vi "Add To DAQmx Task.vi"(6 "Ignore Cal? (F)":bool, 7 "Resistance in":refnum<class "Resistance.lvclass">, 8 "error in (no error)":errorcluster, 9 "Scale Name":string, 10 "Chassis Name":string, 11 "task in":refnum<k21>) -> (0 "error out":errorcluster, 2 "Phys Chan Added":string, 3 "task out":refnum<k21>)   [LabVIEW 2018, in "Measurement Channels.lvlib" / "Resistance.lvclass"]
uses:
  Resistance.lvclass
  C:/Users/Jeff Tipps/Documents/DAQMan/source/Classes/Measurements/Class Channel/Channel.lvclass
  Resistance.lvclass/Resistance.ctl
  Class Channel/Read ChanName.vi
  Class Channel/Read Alias.vi
  Class Channel/Read Scale.vi
  Class Channel/Read Offset.vi
  Class Channel/Read Unit_EU.vi
  <vilib>/DAQmx/create/scale.llb/DAQmx Create Scale (Linear).vi
  <vilib>/DAQmx/create/channels.llb/DAQmx Create Channel (AI-Resistance).vi
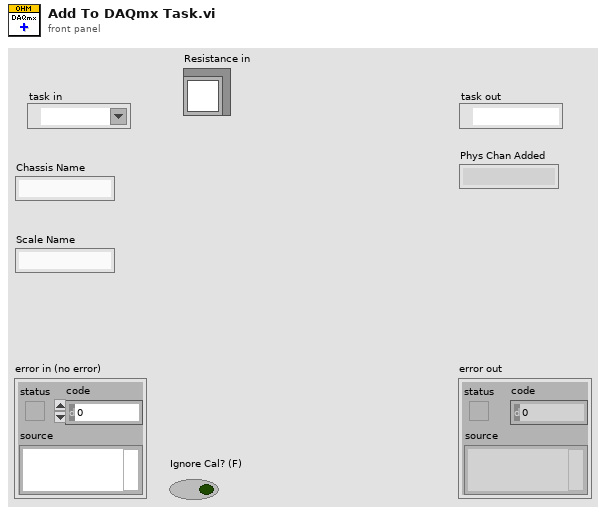
[diagram p1: front panel]
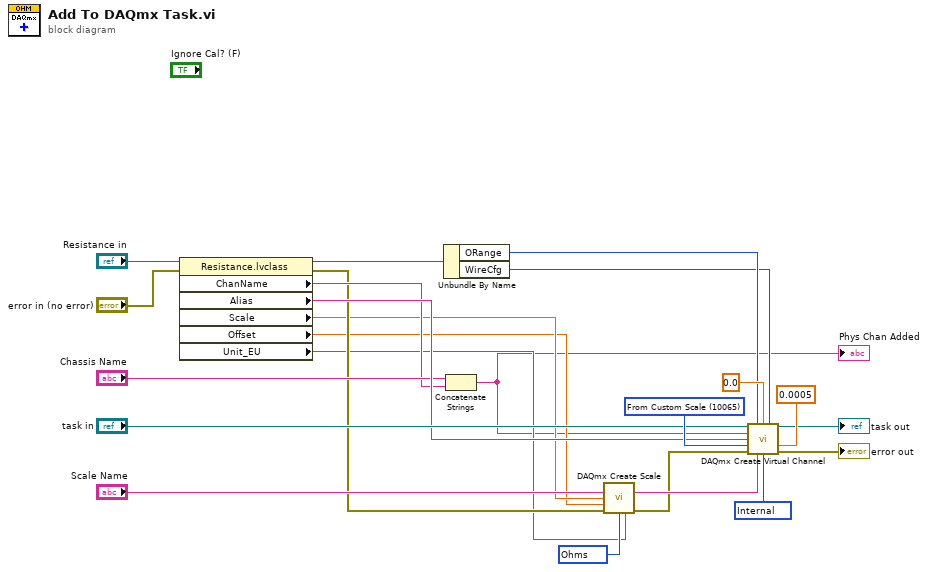
[diagram p0: block diagram]
diagram:
  w22 = 10384 items=["Volts"=10348, "Amps"=10342, "Deg F"=10144, "Deg C"=10143, "Deg R"=10145, "Kelvins"=10325, "Strain"=10299, "Ohms"=10384, "Hz"=10373, "Seconds"=10364, "Meters"=10219, "Inches"=10379, "Degrees"=10146, "Radians"=10273, "Ticks"=10304, "g"=10186, "m/s^2"=12470, "m/s"=15959, "in/s"=15960, "Pascals"=10081, "Newtons"=15875, "Pounds"=15876, "kgf"=15877, "psi"=15879, "bar"=15880, "Nm"=15881, "oz-in"=15882, "lb-in"=15883, "lb-ft"=15884, "Volts/Volt"=15896, "mVolts/Volt"=15897, "From TEDS"=12516] ("pre-scaled units")
  w21 = 10065 items=["Volts"=10348, "From Custom Scale"=10065] ("units")
  w17 = 10200 items=["Internal"=10200, "External"=10167, "None"=10230] ("current excitation source")
  n1 = property class="Resistance.lvclass"(reference="Resistance in", error in="error in (no error)") -> (reference out=w13:refnum<class "Resistance.lvclass">, error out=w7:errorcluster, "ChanName"=w9:string, "Alias"=w11:string, "Scale"=w4:dbl, "Offset"=w3:dbl, "Unit_EU"=w2:string)
  n2 = Unbundle By Name(w13) -> ("ORange"=w19:u16, "WireCfg"=w16:u16)
  n3 = Concatenate Strings("Chassis Name", w9) -> (w1:string)
  "Phys Chan Added" <- w1
  n4 = call-poly <vilib>:"DAQmx Create Scale.vi"("name"="Scale Name", "slope"=w4, "y-intercept"=w3, "error in"=w7, "pre-scaled units"=w22, "scaled units"=w2) -> ("scale out"=w24:tag, "error out"=w23:errorcluster)  [unwired: 8 in]
  n5 = call-poly <vilib>:"DAQmx Create Virtual Channel.vi"("task in"="task in", "maximum value"=w19, "minimum value"=0.0, "resistance configuration"=w16, "physical channels"=w1, "name to assign"=w11, "units"=w21, "current excitation value"=0.0005, "error in"=w23, "custom scale name"=w24, "current excitation source"=w17) -> ("task out"=→"task out":refnum<k21>, "error out"=→"error out":errorcluster)  [unwired: 3 in]
